vi "Sollwert abholen HovaCal.vi"(4 "höchste Konzentration Teilkomponente":dbl, 5 "Einheit in String":string, 6 "Gesamtkonzentration":dbl, 7 "DoIt":bool, 8 "error in (no error)":errorcluster caption="Fehler (Eingang, kein Fehler)", 9 "Punkt":i32, 10 "Sollwert":dbl, 11 "Gasindex":i32) -> (0 "error out":errorcluster caption="Fehler (Ausgang)")   [LabVIEW 2020, in "Linearisierung v2.lvlib"]
uses:
  Linearisierung v2.lvlib
  Aktion Lin Daten aufarbeiten.ctl
  Allgemein/allgemeine Sub-VIs.lvlib
  Gasteiler/Gasteiler.lvlib
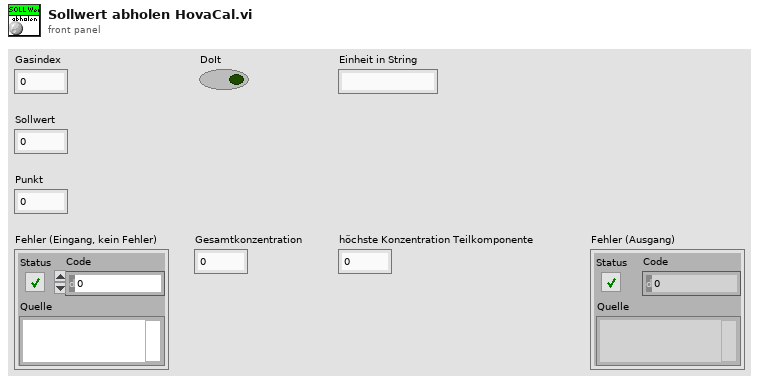
[diagram p1: front panel]
types:
  T1 = typedef "Linearisierung v2.lvlib/Aktion Lin Daten aufarbeiten.ctl" = enum16{"lesen", "Protkolldaten", "speichern", "laden", "EPA auswerten", "Tabelle schreiben", "Lin auswerten", "Tab init", "Stufentabelle", "EPA aktiviert", "Nachbehandlung laden", "Tabelle löschen", "Istwerte löschen", "Zeile löschen", "Zeile einfügen", "LIN aktiviert", "LIN/EPA aktiv laden", "EGAK Tab", "LIN übernehmen", "Tab init ohne Stufen"}
  T2 = typedef "Linearisierung v2.lvlib/Eingabetabelle.ctl" = string[][]
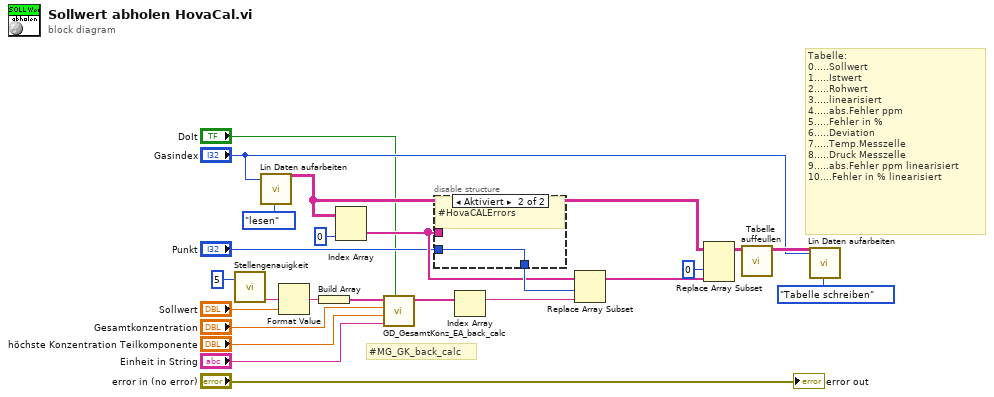
[diagram p0: block diagram]
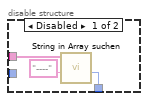
[diagram p2: hidden frame]
diagram:
  # "#MG_GK_back_calc"
  # "Tabelle:\n0.....Sollwert\n1.....Istwert\n2.....Rohwert\n3.....linearisiert\n4.....abs.Fehler ppm\n5.....Fehler in %\n6.....Deviation\n7.....Temp.Messzelle\n8.....Druck Messzelle\n9.....abs.Fehler ppm linearisiert\n10....Fehler in % linearisiert"
  n1 = call "Stellengenauigkeit.vi"("Genauigkeit (6)"=i16 5) -> ("Formatstring"=w21:string)  [unwired: 9 in, 1 out]
  n2 = call "Lin Daten aufarbeiten.vi"("Index (Seite)"="Gasindex", "Aktionen"=Aktion_Lin_Daten_aufarbeiten."lesen") -> ("Eingabetabelle"=w17:T2)  [unwired: 15 in, 10 out]
  n3 = Format Value(format string=w21, value (0)="Sollwert") -> (output string=w4:string)  [unwired: 1 in]
  n4 = Build Array(w4) -> (w2:string[])
  n5 = Index Array(array=w17, index (col)=0 ("Deaktivierter Index (Spalte)")) -> (element=w11:string[])  [unwired: 1 in]
  n6 = call "GD_GesamtKonz_EA_back_calc.vi"("DoIt"="DoIt", "Einheit in String"="Einheit in String", "höchste Konzentration Teilkomponente"="höchste Konzentration Teilkomponente", "Gesamtkonzentration"="Gesamtkonzentration", "Stufentabelle (Eingang)"=w2) -> ("Sollwerte EA Tabelle (Ausgang)"=w3:string[])  [unwired: 6 in]
  n7 = disable-structure shown="Aktiviert" {
    disable-tunnel: [w26 w28] -> w12
    disable-tunnel: w11 -> [w25 _]
    disable-tunnel: "Punkt" -> [_ w28]
    frame Disabled {
      n8 = call "String in Array suchen.vi"("Nach String/Zeichen suchen (-)"="----", "String-Array"=w25) -> ("Index"=w26:i32)  [unwired: 7 in, 2 out]
    }
    frame Enabled {
      # "#HovaCALErrors"
    }
  }
  n9 = Index Array(array=w3) -> (element=w1:string)  [unwired: 1 in]
  n10 = Replace Array Subset(array=w11, new element=w1, index=w12) -> (w5:string[])
  n11 = Replace Array Subset(array=w17, new element=w5, index (col)=0 ("Deaktivierter Index (Spalte)")) -> (w20:T2)  [unwired: 1 in]
  n12 = call "Tabelle auffeullen.vi"("Neue Tabelle"=w20) -> ("Tabelle"=w16:string[][])  [unwired: 10 in]
  n13 = call "Lin Daten aufarbeiten.vi"("Eingabetabelle"=w16, "Index (Seite)"="Gasindex", "Aktionen"=Aktion_Lin_Daten_aufarbeiten."Tabelle schreiben") -> ()  [unwired: 14 in, 11 out]
  "error out" <- "error in (no error)"
